vi "MakePwmCode.vi"() -> (3 "resulting string":string)   [LabVIEW 2023]
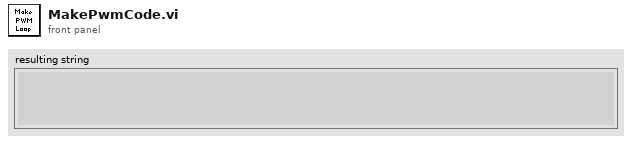
[diagram p1: front panel]
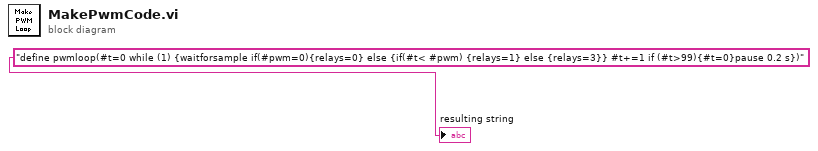
[diagram p0: block diagram]
diagram:
  "resulting string" <- "define pwmloop(#t=0 while (1) {waitforsample if(#pwm=0){relays=0} else {if(#t< #pwm) {relays=1} else {relays=3}} #t+=1 if (#t>99){#t=0}pause 0.2 s})" ("Command")
